vi "Untitled 1.vi"() -> ()   [LabVIEW 2016]
panel:
  out "Komutator":string
  out "Numeric":dbl
  in  "CH4":bool
  in  "CH3":bool
  in  "CH2":bool
  in  "CH1":bool
  in  "max Amplituda":dbl
  out "Ugen":dbl
  in  "Amplituda":dbl
  in  "Iloœæ pomiarów":i32 min=2
  in  "Fk":dbl
  in  "Fp":dbl
  out "Fgen":dbl
  out "Nr pomiaru":dbl
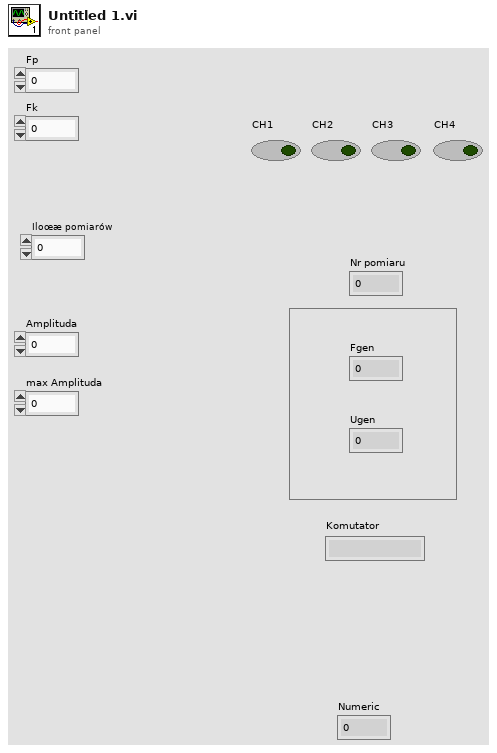
[diagram p1: front panel]
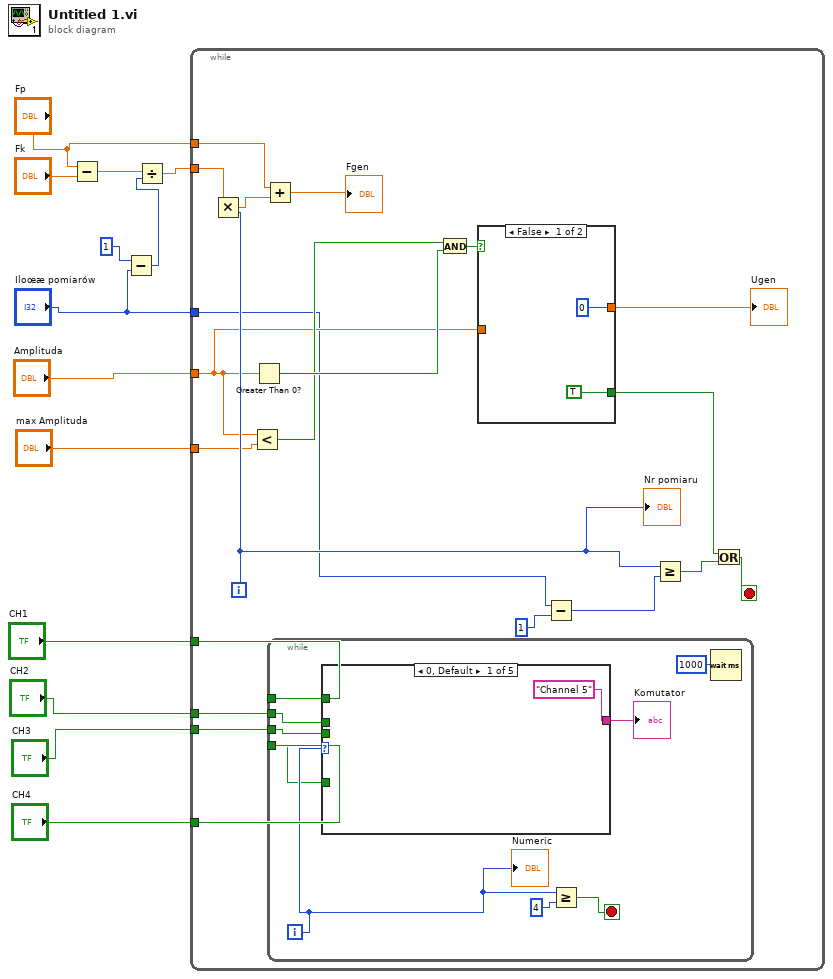
[diagram p0: block diagram]
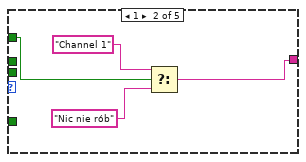
[diagram p2: hidden frame]
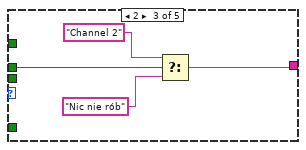
[diagram p3: hidden frame]
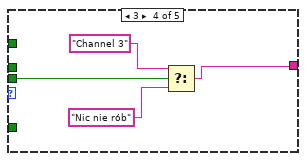
[diagram p4: hidden frame]
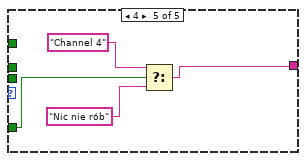
[diagram p5: hidden frame]
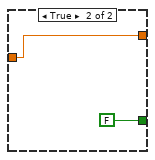
[diagram p6: hidden frame]
diagram:
  n1 = Subtract(x="Fp", y="Fk") -> (x-y=w13:dbl)
  n2 = Subtract(x=1, y="Iloœæ pomiarów") -> (x-y=w11:i32)
  n3 = Divide(x=w13, y=w11) -> (x/y=w10:dbl)
  n4 = while {
    tunnel: "Iloœæ pomiarów" -> [w19]
    tunnel: w10 -> [w34]
    tunnel: "Fp" -> [w21]
    tunnel: "Amplituda" -> [w26]
    tunnel: "max Amplituda" -> [w30]
    tunnel: "CH1" -> [w17]
    tunnel: "CH2" -> [w16]
    tunnel: "CH3" -> [w15]
    tunnel: "CH4" -> [w14]
    i -> [w33]
    stop <- w24 stop-if-true
    n5 = Multiply(x=w34, y=w33) -> (x*y=w32:dbl)
    n6 = Less?(x=w26, y=w30) -> (x < y?=w27:bool)
    n7 = Greater Than 0?(x=w26) -> (x > 0?=w28:bool)
    n8 = Add(x=w21, y=w32) -> (x+y=→"Fgen":dbl)
    n9 = while {
      tunnel: w17 -> [w38]
      tunnel: w16 -> [w37]
      tunnel: w15 -> [w36]
      tunnel: w14 -> [w35]
      i -> [w40]
      stop <- w42 stop-if-true
      n10 = case shown="0, Default" w40 {
        tunnel: ["Channel 5" w45 w49 w54 w57] -> w39
        tunnel: w38 -> [_ w48 _ _ _]
        tunnel: w37 -> [_ _ w50 _ _]
        tunnel: w36 -> [_ _ _ w53 _]
        tunnel: w35 -> [_ _ _ _ w58]
        frame 0, Default {
        }
        frame 1 {
          n11 = Select(t="Channel 1", s=w48, f="Nic nie rób") -> (s? t:f=w45:string)
        }
        frame 2 {
          n12 = Select(t="Channel 2", s=w50, f="Nic nie rób") -> (s? t:f=w49:string)
        }
        frame 3 {
          n13 = Select(t="Channel 3", s=w53, f="Nic nie rób") -> (s? t:f=w54:string)
        }
        frame 4 {
          n14 = Select(t="Channel 4", s=w58, f="Nic nie rób") -> (s? t:f=w57:string)
        }
      }
      "Komutator" <- w39
      n15 = Greater Or Equal?(x=w40, y=4) -> (x >= y?=w42:bool)
      n16 = Wait (ms)(milliseconds to wait=1000) -> ()  [unwired: 1 out]
      "Numeric" <- w40
    }
    n17 = And(x=w27, y=w28) -> (x .and. y?=w29:bool)
    n18 = case shown="False" w29 {
      tunnel: w26 -> [_ w64]
      tunnel: [0 w64] -> w25
      tunnel: [TRUE FALSE] -> w22
      frame False {
      }
      frame True {
      }
    }
    "Ugen" <- w25
    n19 = Subtract(x=w19, y=1) -> (x-y=w18:i32)
    n20 = Greater Or Equal?(x=w33, y=w18) -> (x >= y?=w23:bool)
    n21 = Or(x=w22, y=w23) -> (x .or. y?=w24:bool)
    "Nr pomiaru" <- w33
  }
